vi "Read Ready for iterations.vi"(8 "error in (no error)":errorcluster, 11 "Example Actor in":refnum<class "Example Actor.lvclass">) -> (0 "error out":errorcluster, 2 "Ready for iterations":bool, 3 "Example Actor out":refnum<class "Example Actor.lvclass">)   [LabVIEW 2023, in "Example Iterator NR Actor Implicit Iteration.lvlib" / "Example Actor.lvclass"]
uses:
  Example Actor.lvclass
  Example Actor.lvclass/Example Actor.ctl
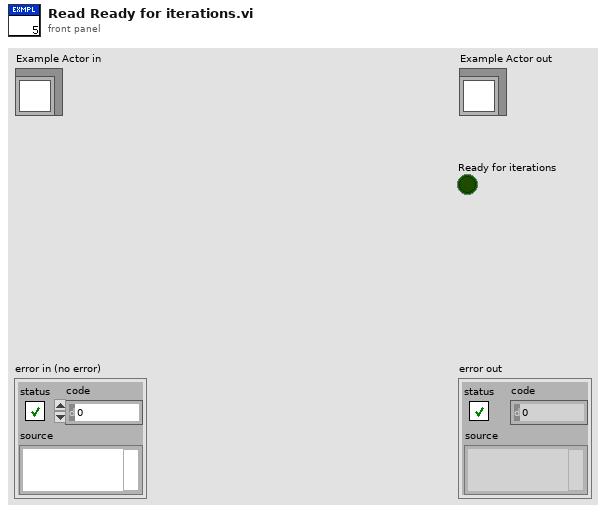
[diagram p1: front panel]
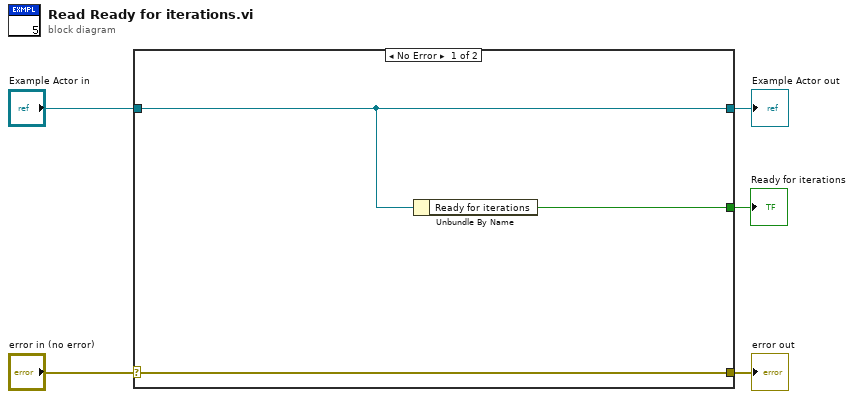
[diagram p0: block diagram]
diagram:
  n1 = case shown="No Error" "error in (no error)" {
    selector: "error in (no error)" -> [w8 w10]
    tunnel: [w8 w10] -> w4
    tunnel: [w7 w9] -> w2
    tunnel: "Example Actor in" -> [w7 w9]
    tunnel: [w6 _] -> w1
    frame No Error {
      n2 = Unbundle By Name(w7) -> ("Ready for iterations"=w6:bool)
    }
    frame Error {
    }
  }
  "error out" <- w4
  "Example Actor out" <- w2
  "Ready for iterations" <- w1
